vi "ORS_GalvoConfig1D_uw.vi"(7 "Force to zero":bool, 8 "error in":errorcluster, 9 "use_digi_trig":bool, 10 "n_triggers":i32=1, 11 "Galvo":T1={"x mirror"="", "y mirror"="", "trig out"="", "x mirror task"="", "y mirror task"="", "trig out task"="", "n_axis"=0, "params"={"n_lines"=512, "n_frames"=1, "force to zero"=FALSE, "Triggers_per_sweep"=0.0, "X center"=0.0, "X span"=0.0, "Y center"=0.0, "Y span"=0.0, "flyb.lines"=0, "n_triggers"=0, "mode"=0, "offset"=5.0, "galvo phase"=0, "span factor"=1.0, "Custom trig."={"n_f to c. trig"=150, "c. trig length"=8, "c. trig interval"=1024, "n_c. trig"=1}, "f_per_pos"=1, "n_dataset"=1, "flyback fr"=1}, "acq trig out"="", "acq trig out task"="", "sample array X"=[], "sample array Y"=[], "custom trig out"="Dev1/port0/line7", "custom trig out task"="", "FDML-box"="TCPIP0::10.153.218.51::23::SOCKET", "ACQ/Galvo"=enum."ADC/FDML", "acq trig out an task"="", "acq trig out an"="", "Galvo Trig input"="", "Galvo Clk input"="", "sample array Acq trig out an"=[]} {"params"."n_dataset" min=1; "params"."X center" format="%^_3g"; "params"."X span" format="%^_3g"; "params"."Y center" format="%^_3g"; "params"."Y span" format="%^_3g"}) -> (0 "error out":errorcluster, 3 "Galvo out":T1={"x mirror"="", "y mirror"="", "trig out"="", "x mirror task"="", "y mirror task"="", "trig out task"="", "n_axis"=0, "params"={"n_lines"=512, "n_frames"=1, "force to zero"=FALSE, "Triggers_per_sweep"=0.0, "X center"=0.0, "X span"=0.0, "Y center"=0.0, "Y span"=0.0, "flyb.lines"=0, "n_triggers"=0, "mode"=0, "offset"=5.0, "galvo phase"=0, "span factor"=1.0, "Custom trig."={"n_f to c. trig"=150, "c. trig length"=8, "c. trig interval"=1024, "n_c. trig"=1}, "f_per_pos"=1, "n_dataset"=1, "flyback fr"=1}, "acq trig out"="", "acq trig out task"="", "sample array X"=[], "sample array Y"=[], "custom trig out"="Dev1/port0/line7", "custom trig out task"="", "FDML-box"="TCPIP0::10.153.218.51::23::SOCKET", "ACQ/Galvo"=enum."ADC/FDML", "acq trig out an task"="", "acq trig out an"="", "Galvo Trig input"="", "Galvo Clk input"="", "sample array Acq trig out an"=[]} {"params"."n_dataset" min=1; "params"."X center" format="%^_3g"; "params"."X span" format="%^_3g"; "params"."Y center" format="%^_3g"; "params"."Y span" format="%^_3g"})   [LabVIEW 2021]
uses:
  Typedefs/ORS_Galvo.ctl
  Typedefs/ORS_Galvo_params.ctl
  <vilib>/DAQmx/create/channels.llb/DAQmx Create Channel (DO-Digital Output).vi
  <vilib>/DAQmx/create/channels.llb/DAQmx Create Channel (AO-Voltage-Basic).vi
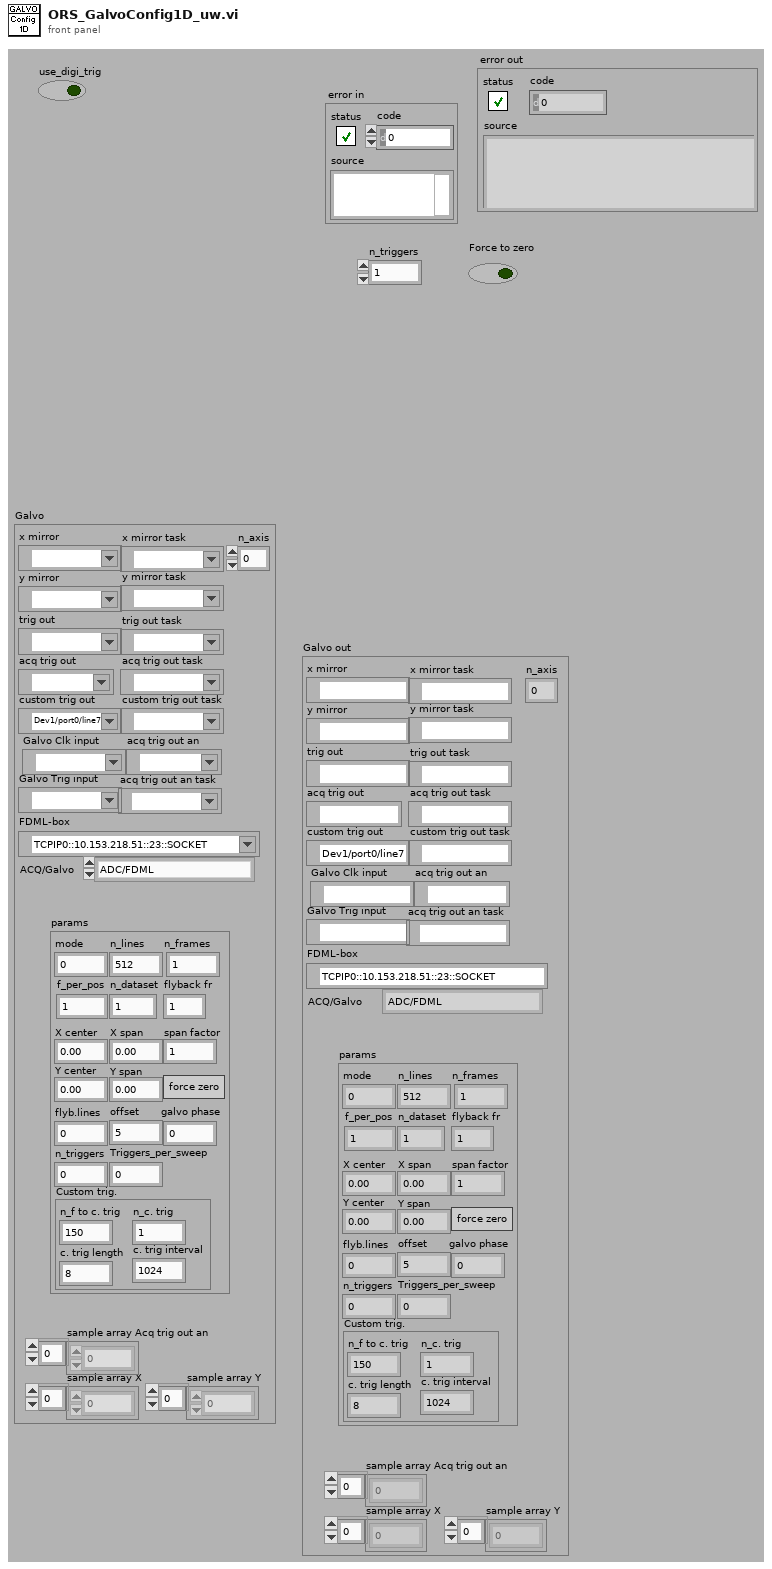
[diagram p1: front panel]
types:
  T1 = typedef "ORS_Galvo.ctl" = cluster{"x mirror":tag, "y mirror":tag, "trig out":tag, "x mirror task":refnum<k21>, "y mirror task":refnum<k21>, "trig out task":refnum<k21>, "n_axis":i32, "params":T2, "acq trig out":tag, "acq trig out task":refnum<k21>, "sample array X":dbl[], "sample array Y":dbl[], "custom trig out":tag, "custom trig out task":refnum<k21>, "FDML-box":refnum<visa-resource-name>, "ACQ/Galvo":enum16{"ADC/FDML", "NI_DAQ", "ADC"}, "acq trig out an task":refnum<k21>, "acq trig out an":tag, "Galvo Trig input":tag, "Galvo Clk input":tag, "sample array Acq trig out an":dbl[]}
  T2 = typedef "ORS_Galvo_params.ctl" = cluster{"n_lines":i32, "n_frames":i32, "force to zero":bool, "Triggers_per_sweep":dbl, "X center":dbl, "X span":dbl, "Y center":dbl, "Y span":dbl, "flyb.lines":i32, "n_triggers":i32, "mode":i32, "offset":dbl, "galvo phase":i32, "span factor":dbl, "Custom trig.":cluster{"n_f to c. trig":i32, "c. trig length":i32, "c. trig interval":i32, "n_c. trig":i32}, "f_per_pos":i32, "n_dataset":u32, "flyback fr":u16}
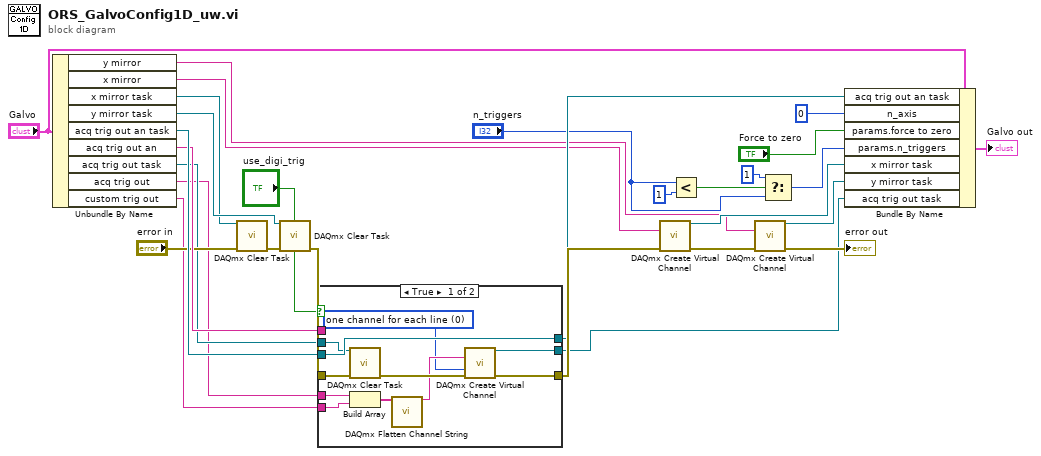
[diagram p0: block diagram]
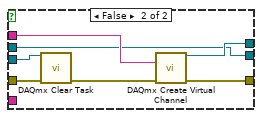
[diagram p2: hidden frame]
diagram:
  n1 = Unbundle By Name("Galvo") -> ("y mirror"=w13:tag, "x mirror"=w15:tag, "x mirror task"=w9:refnum<k21>, "y mirror task"=w20:refnum<k21>, "acq trig out an task"=w22:refnum<k21>, "acq trig out an"=w21:tag, "acq trig out task"=w4:refnum<k21>, "acq trig out"=w2:tag, "custom trig out"=w1:tag)
  n2 = call <vilib>:"DAQmx Clear Task.vi"("task in"=w9, "error in"="error in") -> ("error out"=w19:errorcluster)  [unwired: 13 in]
  n3 = call <vilib>:"DAQmx Clear Task.vi"("task in"=w20, "error in"=w19) -> ("error out"=w18:errorcluster)  [unwired: 13 in]
  n4 = case shown="True" "use_digi_trig" {
    tunnel: w22 -> [w40 w47]
    tunnel: w21 -> [_ w46]
    tunnel: w18 -> [w38 w45]
    tunnel: [w37 w44] -> w17
    tunnel: [w40 w43] -> w16
    tunnel: w4 -> [w36 w41]
    tunnel: [w31 w41] -> w3
    tunnel: w2 -> [w35 _]
    tunnel: w1 -> [w34 _]
    frame True {
      w30 = 0 items=["one channel for each line", "one channel for all lines"] ("line grouping")
      n5 = call <vilib>:"DAQmx Clear Task.vi"("task in"=w36, "error in"=w38) -> ("error out"=w39:errorcluster)  [unwired: 13 in]
      n6 = Build Array(w35, w34) -> (w33:tag[])
      n7 = call <vilib>:"DAQmx Flatten Channel String.vi"("names in"=w33) -> ("names out"=w32:string)  [unwired: 13 in, 1 out]
      n8 = call-poly <vilib>:"DAQmx Create Virtual Channel.vi"("lines"=w32, "line grouping"=w30, "error in"=w39) -> ("task out"=w31:refnum<k21>, "error out"=w37:errorcluster)  [unwired: 11 in]
    }
    frame False {
      n9 = call <vilib>:"DAQmx Clear Task.vi"("task in"=w47, "error in"=w45) -> ("error out"=w42:errorcluster)  [unwired: 13 in]
      n10 = call-poly <vilib>:"DAQmx Create Virtual Channel.vi"("physical channels"=w46, "error in"=w42) -> ("task out"=w43:refnum<k21>, "error out"=w44:errorcluster)  [unwired: 12 in]
    }
  }
  n11 = call-poly <vilib>:"DAQmx Create Virtual Channel.vi"("physical channels"=w15, "error in"=w17) -> ("task out"=w14:refnum<k21>, "error out"=w10:errorcluster)  [unwired: 12 in]
  n12 = Less?(x="n_triggers", y=1) -> (x < y?=w27:bool)
  n13 = call-poly <vilib>:"DAQmx Create Virtual Channel.vi"("physical channels"=w13, "error in"=w10) -> ("task out"=w12:refnum<k21>, "error out"=→"error out":errorcluster)  [unwired: 12 in]
  n14 = Select(t=1 ("n_triggers"), s=w27, f="n_triggers") -> (s? t:f=w26:i32)
  n15 = Bundle By Name(cluster="Galvo", "acq trig out an task"=w16, "n_axis"=0, "params.force to zero"="Force to zero", "params.n_triggers"=w26, "x mirror task"=w14, "y mirror task"=w12, "acq trig out task"=w3) -> (→"Galvo out":T1)
